vi "test_mode_control.vi"(2 "test mode":string[](array[string])) -> (6 "test mode str out":string)   [LabVIEW 2015]
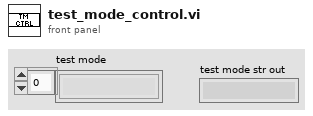
[diagram p1: front panel]
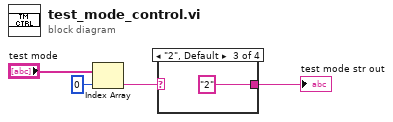
[diagram p0: block diagram]
diagram:
  n1 = Index Array(array="test mode", index=0) -> (element=w1:string)
  n2 = case shown="\"2\", Default" w1 {
    selector: w1 -> [w5 w6 _ w8]
    tunnel: [w5 w6 "2" w8] -> w4
    frame "0" {
    }
    frame "1" {
    }
    frame "2", Default {
    }
    frame "3" {
    }
  }
  "test mode str out" <- w4
